vi "LIN Read.vi"(7 "Len":u32, 9 "pLINMsg":T1, 10 "LINIndex":u8, 11 "DevHandle":i32) -> (1 "pLINMsg out":T1, 3 "function return":i32)   [LabVIEW 2010, in "usb2lin.lvlib"]
doc: "int WINAPI LIN_Read(int DevHandle,unsigned char LINIndex,LIN_MSG *pLINMsg,unsigned int Len);"
uses:
  usb2lin.lvlib
  USB2XXX/trunk/USB2XXX/USB2XXX/vs2010/Release/USB2XXX.dll
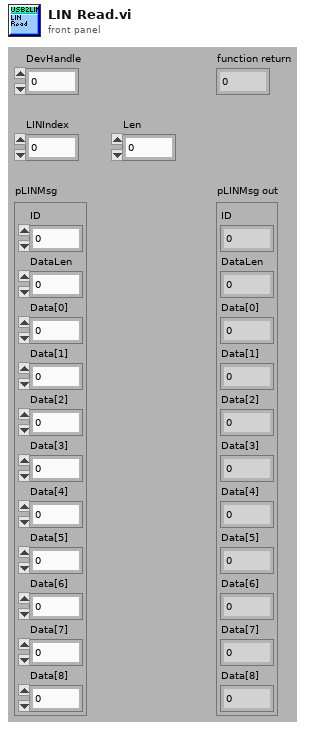
[diagram p1: front panel]
types:
  T1 = cluster{"ID":u8, "DataLen":u8, "Data[0]":u8, "Data[1]":u8, "Data[2]":u8, "Data[3]":u8, "Data[4]":u8, "Data[5]":u8, "Data[6]":u8, "Data[7]":u8, "Data[8]":u8}
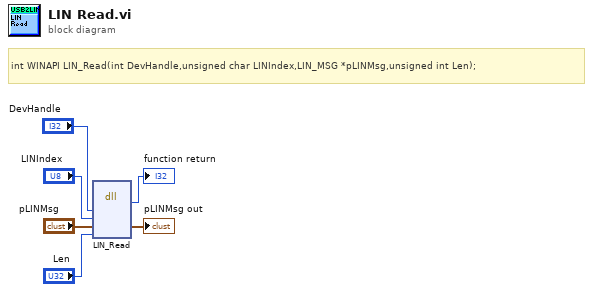
[diagram p0: block diagram]
diagram:
  # "int WINAPI LIN_Read(int DevHandle,unsigned char LINIndex,LIN_MSG *pLINMsg,unsigned int Len);"
  n1 = dll-call lib="E:/OtherWork/STM32/USB2XXX/trunk/USB2XXX/USB2XXX/vs2010/Release/USB2XXX.*" fn="LIN_Read"("DevHandle"="DevHandle", "LINIndex"="LINIndex", "pLINMsg"="pLINMsg", "Len"="Len") -> (→"function return":i32, "pLINMsg"=→"pLINMsg out":T1)  [unwired: 6 in, 2 out]
